vi "Rotating Vectors.vi"() -> ()   [LabVIEW 2019]
uses:
  <vilib>/Analysis/1siggen.llb/Ramp Pattern by Samples.vi
  <vilib>/Analysis/2dsp.llb/Complex FFT.vi
  <vilib>/Analysis/2dsp.llb/Real FFT.vi
  Sub - Arrow Point Calculate.vi
  <vilib>/Analysis/NI_AALPro.lvlib
  <vilib>/Analysis/NI_AALBase.lvlib
panel:
  in  "Message Amplitude":dbl=0.5
  in  "DC Offset":dbl
  in  "RF Frequency":dbl
  in  "Message Frequency":dbl=0.2 step=0.1
  in  "stop":bool
  in  "vi path":path
  in  "Vertical Load Button":bool
  in  "Vertical Pause Button":bool
  in  "Upconvert Baseband":bool=TRUE
  out "Vector Graph":cluster{"z vector":cdb[]}[](graph)=[{"z vector"=[0.0+0.0i, 0.20656463842372266-0.4553361946439979i, 0.21632021300842424-0.355813188436778i, 0.20656463842372266-0.4553361946439979i, 0.12525297407962463-0.3971261161215226i, 0.20656463842372266-0.4553361946439979i]}, {"z vector"=[0.0+0.0i, 0.20656463842372266+0.4553361946439979i, 0.1252529740796247+0.3971261161215225i, 0.20656463842372266+0.4553361946439979i, 0.21632021300842427+0.355813188436778i, 0.20656463842372266+0.4553361946439979i]}, {"z vector"=[0.0+0.0i, 0.4131292768474453+0.0i, 0.32652673646900143+0.05000000000000002i, 0.4131292768474453+0.0i, 0.3265267364690015-0.050000000000000044i, 0.4131292768474453+0.0i]}, {"z vector"=[0.0+0.0i, 0.0+0.0i, nan+nani, 0.0+0.0i, nan+nani, 0.0+0.0i]}, {"z vector"=[0.0+0.0i, 0.4131292768474453+0.0i, 0.32652673646900143+0.05000000000000002i, 0.4131292768474453+0.0i, 0.3265267364690015-0.050000000000000044i, 0.4131292768474453+0.0i]}, {"z vector"=[0.0+0.0i, 0.4131292768474453+0.0i, 0.32652673646900143+0.05000000000000002i, 0.4131292768474453+0.0i, 0.3265267364690015-0.050000000000000044i, 0.4131292768474453+0.0i]}, {"z vector"=[0.4131292768474453+0.0i, 0.4131292768474453+0.0i, nan+nani, 0.4131292768474453+0.0i, nan+nani, 0.4131292768474453+0.0i]}, {"z vector"=[0.0+0.0i, 1.0+0.0i, 0.9133974596215562+0.05000000000000002i, 1.0+0.0i, 0.9133974596215562-0.050000000000000044i, 1.0+0.0i]}]
  out "Time Domain":cluster{dbl, dbl, dbl}(graph)={0.4131292768474453, 0.4131292768474453, 1.0}
  out "Vector Sum Frequency Response":dbl[][](graph)
  out "Individual Vectors":dbl[][](graph)
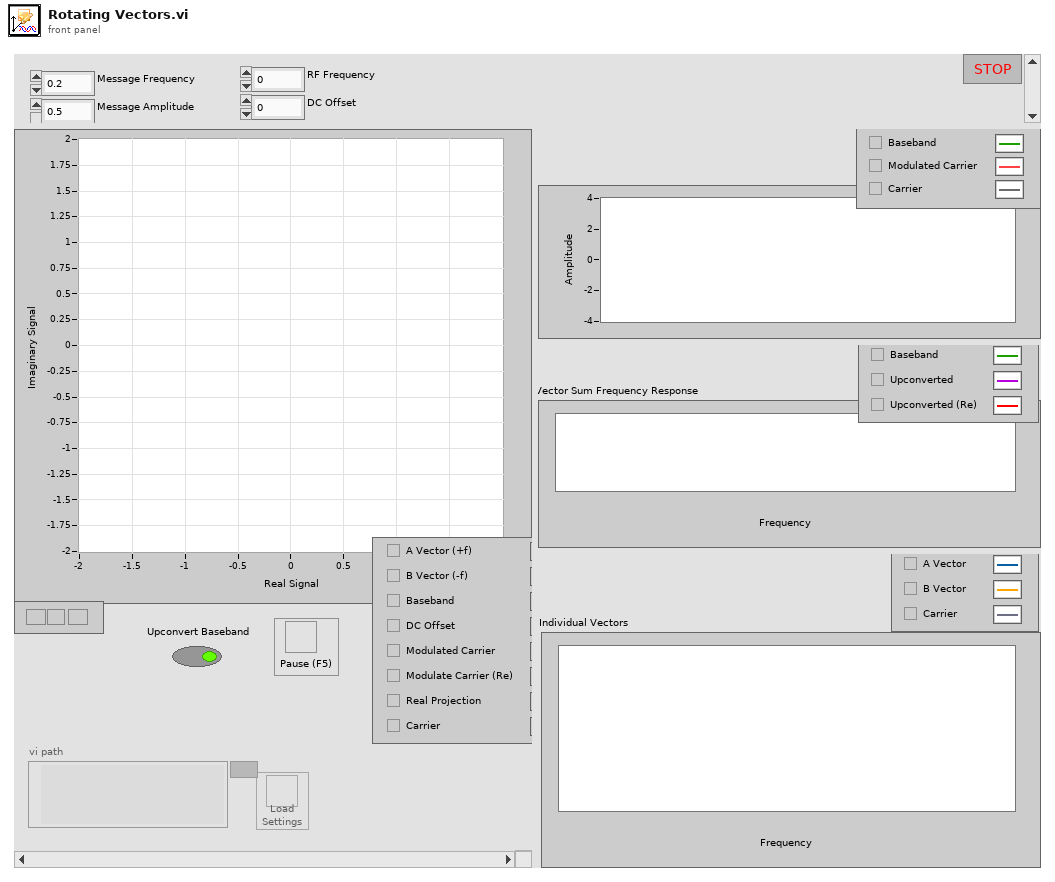
[diagram p1: front panel]
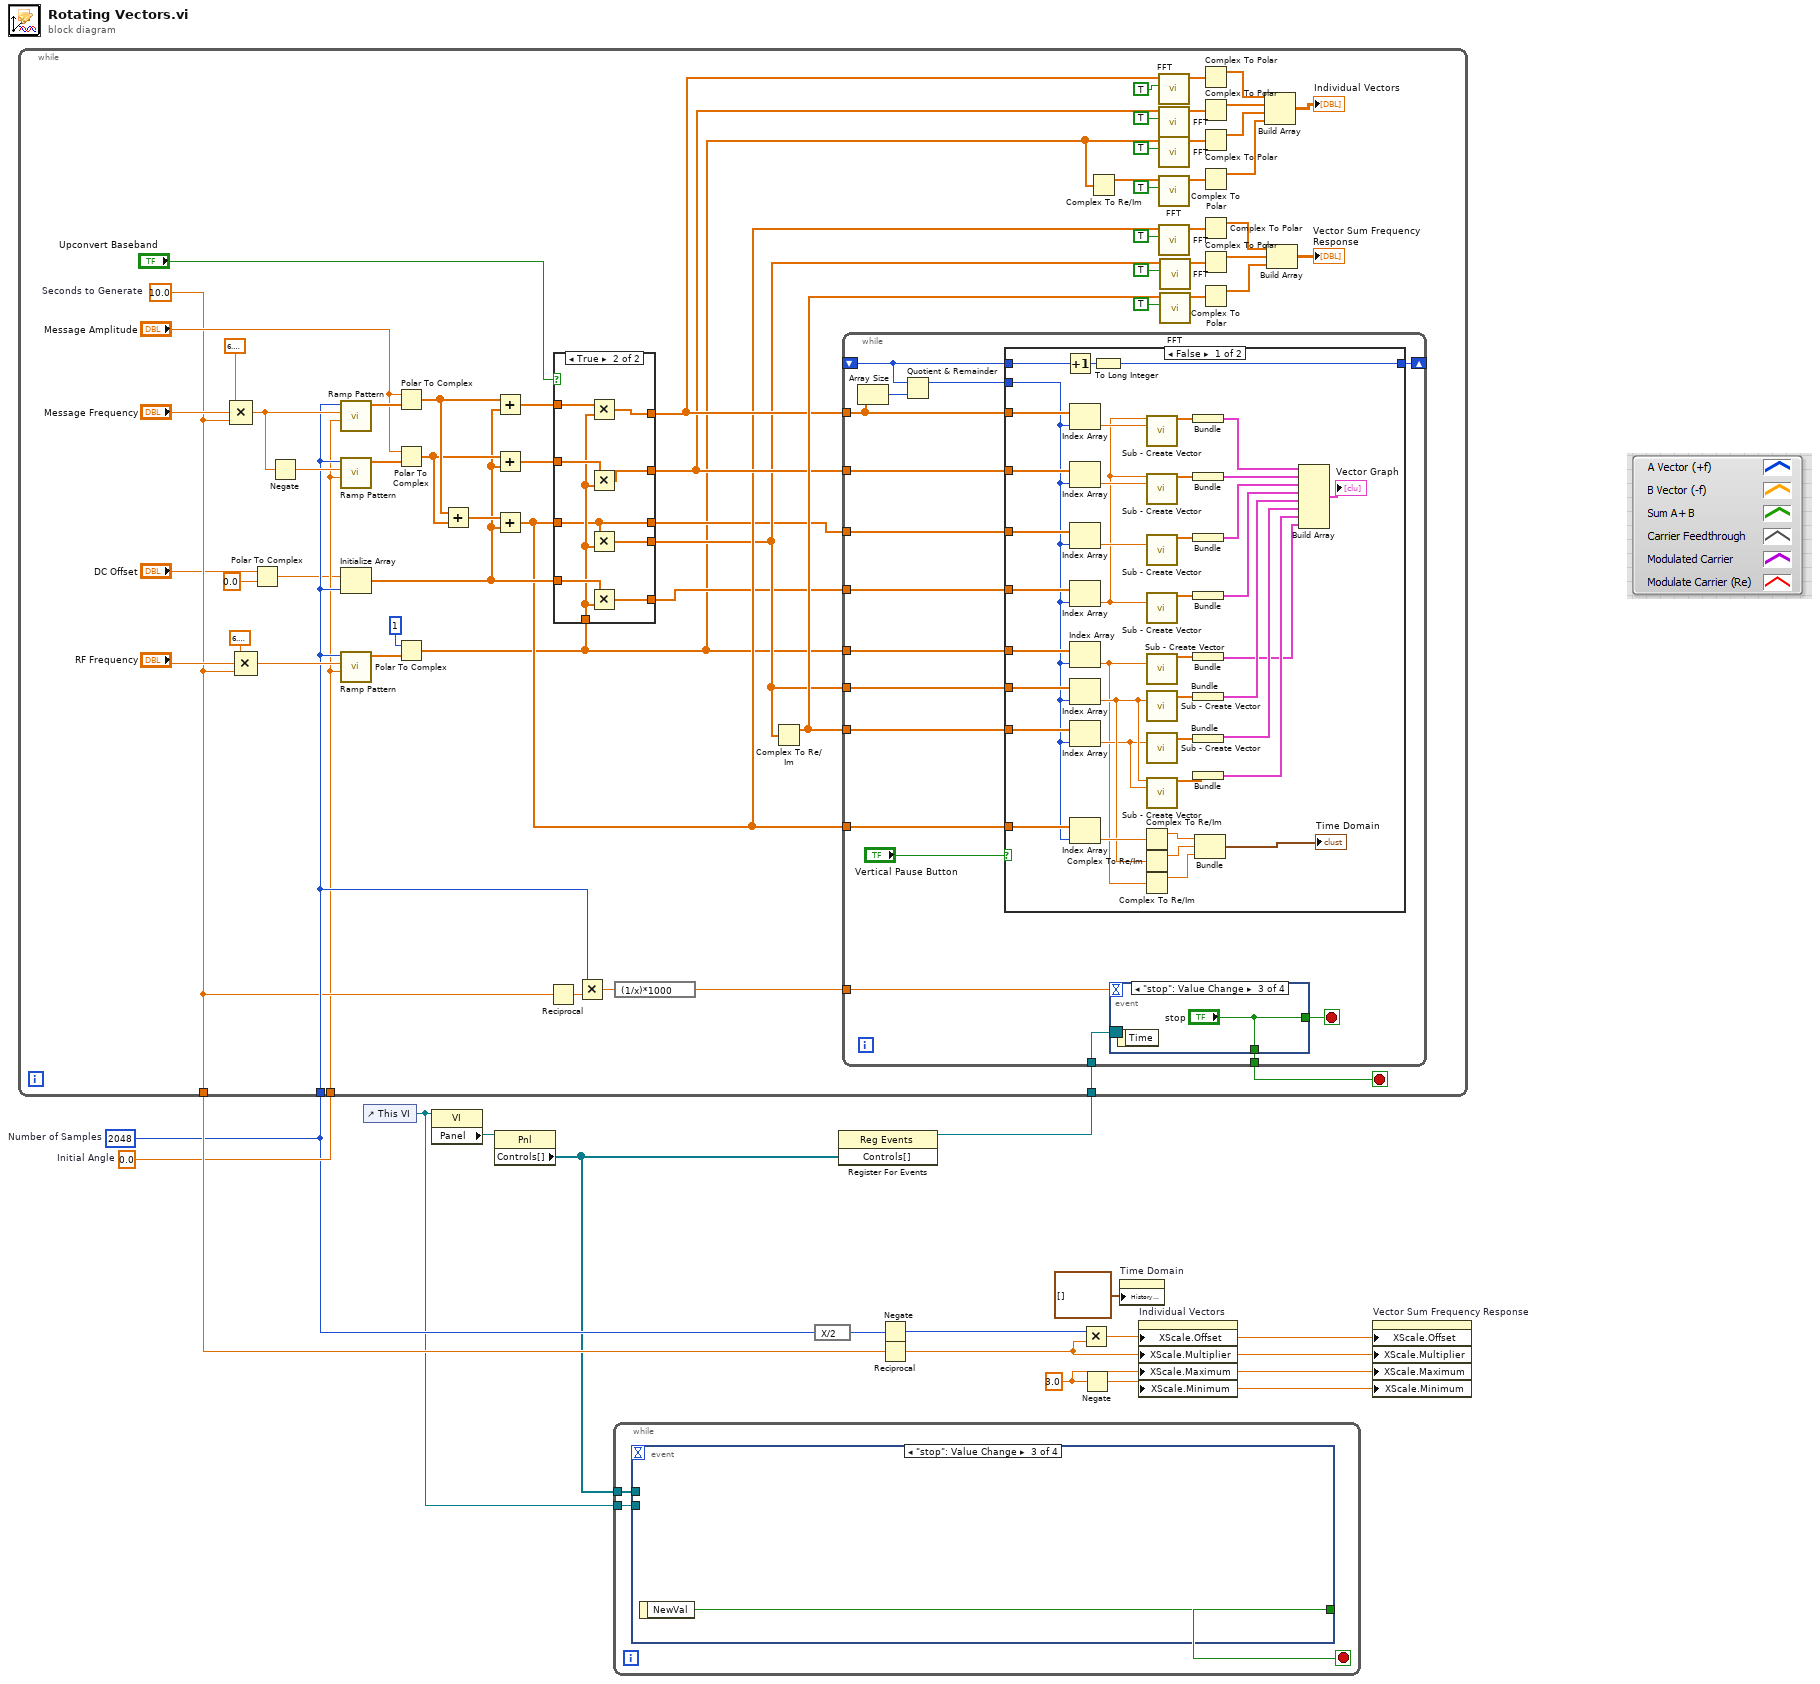
[diagram p0: block diagram]
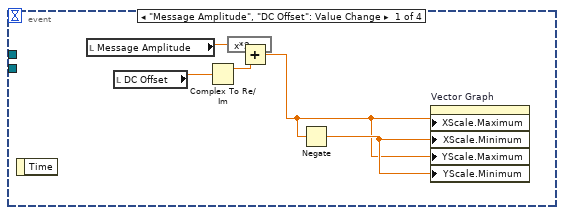
[diagram p2: hidden frame]
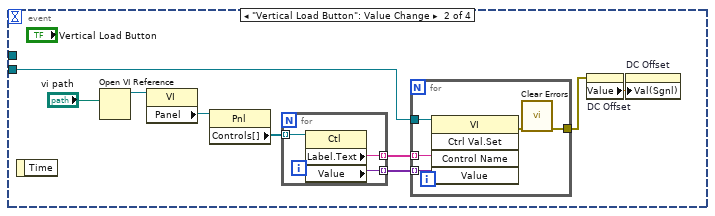
[diagram p3: hidden frame]
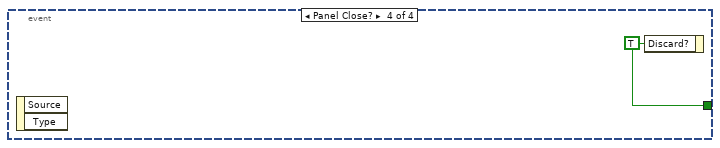
[diagram p4: hidden frame]
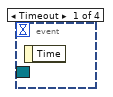
[diagram p7: hidden frame]
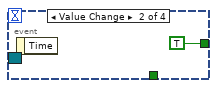
[diagram p8: hidden frame]
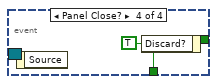
[diagram p9: hidden frame]
diagram:
  w4 = 2048  # Number of Samples
  w5 = 0.0  # Initial Angle
  w11 = 3.0 ("X Scale.Range:Maximum")
  n1 = control-ref of="This VI"() -> (w1:refnum<vi>)
  n2 = property class="VI"(reference=w1) -> ("Panel"=w7:refnum<vi>)  [unwired: 1 in, 2 out]
  n3 = property class="Pnl"(reference=w7) -> ("Controls[]"=w2:refnum<vi>[])  [unwired: 1 in, 2 out]
  n4 = while {
    tunnel: w2 -> [w16]
    tunnel: w1 -> [w15]
    stop <- w17 stop-if-true
    n5 = event shown="[2] \"stop\": Value Change" {
      selector: _ -> [_ _ _ _]
      dyn-events: _ -> [_ _ _ _]
      timeout: _ -> [_ _ _ _]
      tunnel: [_ _ w41 w42] -> w17
      tunnel: w16 -> [_ _ _ _]
      tunnel: w15 -> [_ w29 _ _]
      event "Message Amplitude", "DC Offset": Value Change {
        n6 = event-data() -> ()  [unwired: 1 in, 1 out]
        n7 = local read "Message Amplitude"() -> (w21:dbl)
        n8 = local read "DC Offset"() -> (w22:dbl)
        n9 = Complex To Re/Im(x + iy=w22) -> (x=w19:dbl)  [unwired: 1 out]
        n10 = expression code="x*2"(w21) -> (w18:dbl)
        n11 = Add(x=w18, y=w19) -> (x+y=w20:dbl)
        n12 = Negate(x=w20) -> (-x=w23:dbl)
        n13 = property on="Vector Graph" class="XYGraph (strict)"("XScale.Maximum"=w20, "XScale.Minimum"=w23, "YScale.Maximum"=w20, "YScale.Minimum"=w23) -> ()  [unwired: 2 in, 2 out]
      }
      event "Vertical Load Button": Value Change {
        n14 = event-data() -> ()  [unwired: 1 in, 1 out]
        n15 = Open VI Reference(vi path="vi path") -> (vi reference=w31:refnum<vi>)  [unwired: 5 in, 1 out]
        n16 = property class="VI"(reference=w31) -> ("Panel"=w32:refnum<vi>)  [unwired: 1 in, 2 out]
        n17 = property class="Pnl"(reference=w32) -> ("Controls[]"=w30:refnum<vi>[])  [unwired: 1 in, 2 out]
        n18 = for {
          tunnel: w30 -> [w40] mode=indexing
          tunnel: [w39] -> w28 mode=indexing
          tunnel: [w38] -> w27 mode=indexing
          n19 = property class="Ctl"(reference=w40) -> ("Label.Text"=w39:string, "Value"=w38:variant)  [unwired: 1 in, 2 out]
        }
        n20 = for {
          tunnel: w29 -> [w37]
          tunnel: w28 -> [w36] mode=indexing
          tunnel: w27 -> [w35] mode=indexing
          tunnel: [w33] -> w24
          n21 = invoke class="VI" method="Ctrl Val.Set"(reference=w37, "Control Name"=w36, "Value"=w35) -> (error out=w34:errorcluster)  [unwired: 2 in, 4 out]
          n22 = call <vilib>:"Clear Errors.vi"("error in (no error)"=w34) -> ("error out"=w33:errorcluster)  [unwired: 5 in, 1 out]
        }
        n23 = property on="DC Offset" class="DigNum (strict)"(error in=w24) -> ("Value"=w25:dbl)  [unwired: 1 in, 2 out]
        n24 = property on="DC Offset" class="DigNum (strict)"("Val(Sgnl)"=w25) -> ()  [unwired: 2 in, 2 out]
      }
      event "stop": Value Change {
        n25 = event-data() -> ("NewVal"=w41:bool)  [unwired: 1 in]
      }
      event Panel Close? {
        w42 = TRUE ("Discard?")
        n26 = event-data() -> ()  [unwired: 1 in, 2 out]
        n27 = event-data("Discard?"=w42) -> ()  [unwired: 1 in, 1 out]
      }
    }
  }
  n28 = expression code="X/2"(w4) -> (w13:i32)
  n29 = register-events(w2) -> (reference out=w6:refnum<event-registration>)  [unwired: 2 in, 1 out]
  n30 = while {
    tunnel: [w72] -> w8
    tunnel: w4 -> [w76]
    tunnel: w6 -> [w75]
    tunnel: w5 -> [w65]
    stop <- w73 stop-if-true
    w72 = 10.0  # Seconds to Generate
    n31 = Compound Arithmetic op=MULTIPLY(6.283185307179586, "Message Frequency", w72) -> (w85:dbl)
    n32 = Compound Arithmetic op=MULTIPLY(6.283185307179586, "RF Frequency", w72) -> (w79:dbl)
    n33 = Polar To Complex(1:0.0 ("theta"), 2:"DC Offset") -> (0:w51:cdb)
    n34 = Negate(x=w85) -> (-x=w87:dbl)
    n35 = call-poly <vilib>:"Ramp Pattern.vi"("start"=w65, "end"=w85, "samples"=w76) -> ("Ramp Pattern"=w98:dbl[])  [unwired: 7 in, 1 out]
    n36 = call-poly <vilib>:"Ramp Pattern.vi"("start"=w65, "end"=w87, "samples"=w76) -> ("Ramp Pattern"=w88:dbl[])  [unwired: 7 in, 1 out]
    n37 = Initialize Array(w51, w76) -> (w55:cdb[])
    n38 = call-poly <vilib>:"Ramp Pattern.vi"("start"=w65, "end"=w79, "samples"=w76) -> ("Ramp Pattern"=w86:dbl[])  [unwired: 7 in, 1 out]
    n39 = Polar To Complex(1:w98, 2:"Message Amplitude") -> (0:w78:cdb[])
    n40 = Polar To Complex(1:w88, 2:"Message Amplitude") -> (0:w77:cdb[])
    n41 = Polar To Complex(1:w86, 2:1) -> (0:w45:cdb[])
    n42 = Add(x=w78, y=w77) -> (x+y=w66:cdb[])
    n43 = Add(x=w78, y=w55) -> (x+y=w60:cdb[])
    n44 = Add(x=w77, y=w55) -> (x+y=w59:cdb[])
    n45 = Add(x=w66, y=w55) -> (x+y=w54:cdb[])
    n46 = Reciprocal(x=w72) -> (1/x=w96:dbl)
    n47 = case shown="True" "Upconvert Baseband" {
      tunnel: w60 -> [w106 w117]
      tunnel: w59 -> [w107 w116]
      tunnel: w55 -> [w108 w115]
      tunnel: w54 -> [w105 w109]
      tunnel: w45 -> [_ w114]
      tunnel: [w108 w113] -> w48
      tunnel: [w105 w112] -> w53
      tunnel: [w107 w111] -> w56
      tunnel: [w106 w110] -> w57
      tunnel: [w105 w109] -> w49
      frame False {
      }
      frame True {
        n48 = Multiply(x=w117, y=w114) -> (x*y=w110:cdb[])
        n49 = Multiply(x=w116, y=w114) -> (x*y=w111:cdb[])
        n50 = Multiply(x=w109, y=w114) -> (x*y=w112:cdb[])
        n51 = Multiply(x=w115, y=w114) -> (x*y=w113:cdb[])
      }
    }
    n52 = Multiply(x=w76, y=w96) -> (x*y=w97:dbl)
    n53 = expression code="(1/x)*1000"(w97) -> (w104:dbl)
    n54 = Complex To Re/Im(x + iy=w53) -> (x=w61:dbl[])  [unwired: 1 out]
    n55 = while {
      tunnel: w57 -> [w125]
      tunnel: w104 -> [w130]
      tunnel: w56 -> [w134]
      tunnel: w49 -> [w133]
      tunnel: w53 -> [w132]
      tunnel: w48 -> [w131]
      tunnel: w75 -> [w126]
      tunnel: [w128] -> w73
      tunnel: w61 -> [w127]
      tunnel: w54 -> [w123]
      shift-right: [w120] -> _
      shift-left: _ -> [w121]
      tunnel: w45 -> [w118]
      stop <- w129 stop-if-true
      n56 = Array Size(array=w125) -> (size(s)=w124:i32)
      n57 = Quotient & Remainder(x=w121, y=w124) -> (x-y*floor(x/y)=w122:i32)  [unwired: 1 out]
      n58 = case shown="False" "Vertical Pause Button" {
        tunnel: w134 -> [w172 _]
        tunnel: w133 -> [w167 _]
        tunnel: w132 -> [w166 _]
        tunnel: w131 -> [w161 _]
        tunnel: w127 -> [w158 _]
        tunnel: w125 -> [w156 _]
        tunnel: w123 -> [w151 _]
        tunnel: w122 -> [w137 _]
        tunnel: w121 -> [w147 w176]
        tunnel: [w146 w176] -> w120
        tunnel: w118 -> [w139 _]
        frame False {
          n59 = Increment(x=w147) -> (x+1=w145:i32)
          n60 = Index Array(array=w156, index=w137) -> (element=w153:cdb)
          n61 = Index Array(array=w172, index=w137) -> (element=w154:cdb)
          n62 = Index Array(array=w167, index=w137) -> (element=w155:cdb)
          n63 = Index Array(array=w161, index=w137) -> (element=w152:cdb)
          n64 = Index Array(array=w139, index=w137) -> (element=w136:cdb)
          n65 = Index Array(array=w166, index=w137) -> (element=w142:cdb)
          n66 = Index Array(array=w158, index=w137) -> (element=w141:dbl)
          n67 = Index Array(array=w151, index=w137) -> (element=w150:cdb)
          n68 = To Long Integer(number=w145) -> (32bit integer=w146:i32)
          n69 = Complex To Re/Im(x + iy=w150) -> (x=w165:dbl)  [unwired: 1 out]
          n70 = Complex To Re/Im(x + iy=w142) -> (x=w164:dbl)  [unwired: 1 out]
          n71 = Complex To Re/Im(x + iy=w136) -> (x=w135:dbl)  [unwired: 1 out]
          n72 = call "Sub - Create Vector.vi"("Vector Start (0 +0i)"=w152, "Vector End"=w153) -> ("Vector Points"=w171:cdb[])  [unwired: 13 in]
          n73 = call "Sub - Create Vector.vi"("Vector Start (0 +0i)"=w152, "Vector End"=w154) -> ("Vector Points"=w170:cdb[])  [unwired: 13 in]
          n74 = call "Sub - Create Vector.vi"("Vector End"=w155) -> ("Vector Points"=w168:cdb[])  [unwired: 14 in]
          n75 = call "Sub - Create Vector.vi"("Vector End"=w152) -> ("Vector Points"=w162:cdb[])  [unwired: 14 in]
          n76 = call "Sub - Create Vector.vi"("Vector End"=w136) -> ("Vector Points"=w140:cdb[])  [unwired: 14 in]
          n77 = call "Sub - Create Vector.vi"("Vector End"=w142) -> ("Vector Points"=w159:cdb[])  [unwired: 14 in]
          n78 = call "Sub - Create Vector.vi"("Vector End"=w141) -> ("Vector Points"=w157:cdb[])  [unwired: 14 in]
          n79 = call "Sub - Create Vector.vi"("Vector Start (0 +0i)"=w142, "Vector End"=w141) -> ("Vector Points"=w144:cdb[])  [unwired: 13 in]
          n80 = Bundle("Vector Points"=w171) -> (w175:cluster{"Vector Points":cdb[]})  [unwired: 1 in]
          n81 = Bundle("Vector Points"=w170) -> (w173:cluster{"Vector Points":cdb[]})  [unwired: 1 in]
          n82 = Bundle("Vector Points"=w168) -> (w169:cluster{"Vector Points":cdb[]})  [unwired: 1 in]
          n83 = Bundle("Vector Points"=w162) -> (w160:cluster{"Vector Points":cdb[]})  [unwired: 1 in]
          n84 = Bundle("Vector Points"=w140) -> (w138:cluster{"Vector Points":cdb[]})  [unwired: 1 in]
          n85 = Bundle("Vector Points"=w159) -> (w149:cluster{"Vector Points":cdb[]})  [unwired: 1 in]
          n86 = Bundle("Vector Points"=w157) -> (w148:cluster{"Vector Points":cdb[]})  [unwired: 1 in]
          n87 = Bundle("Vector Points"=w144) -> (w143:cluster{"Vector Points":cdb[]})  [unwired: 1 in]
          n88 = Bundle(w165, w164, w135) -> (→"Time Domain":cluster{dbl, dbl, dbl})  [unwired: 1 in]
          n89 = Build Array(w175, w173, w169, w160, w149, w148, w143, w138) -> (→"Vector Graph":cluster{"Vector Points":cdb[]}[])
        }
        frame True {
        }
      }
      n90 = event shown="[2] \"stop\": Value Change" {
        selector: w126 -> [_ _ _ _]
        dyn-events: _ -> [_ _ _ _]
        timeout: w130 -> [_ _ _ _]
        tunnel: [_ TRUE "stop" w179] -> w129
        tunnel: [_ _ "stop" w179] -> w128
        event Timeout {
          n91 = event-data() -> ()  [unwired: 1 in, 1 out]
        }
        event Value Change {
          n92 = event-data() -> ()  [unwired: 1 in, 1 out]
        }
        event "stop": Value Change {
          n93 = event-data() -> ()  [unwired: 1 in, 1 out]
        }
        event Panel Close? {
          w179 = TRUE ("Discard?")
          n94 = event-data() -> ()  [unwired: 1 in, 1 out]
          n95 = event-data("Discard?"=w179) -> ()  [unwired: 1 in, 1 out]
        }
      }
    }
    n96 = Complex To Re/Im(x + iy=w45) -> (x=w44:dbl[])  [unwired: 1 out]
    n97 = call-poly <vilib>:"FFT.vi"("shift?"=TRUE, "X"=w57) -> ("FFT {X}"=w102:cdb[])  [unwired: 8 in, 1 out]
    n98 = call-poly <vilib>:"FFT.vi"("shift?"=TRUE, "X"=w56) -> ("FFT {X}"=w95:cdb[])  [unwired: 8 in, 1 out]
    n99 = call-poly <vilib>:"FFT.vi"("shift?"=TRUE, "X"=w45) -> ("FFT {X}"=w69:cdb[])  [unwired: 8 in, 1 out]
    n100 = call-poly <vilib>:"FFT.vi"("shift?"=TRUE, "X"=w44) -> ("FFT {X}"=w47:cdb[])  [unwired: 8 in, 1 out]
    n101 = call-poly <vilib>:"FFT.vi"("shift?"=TRUE, "X"=w54) -> ("FFT {X}"=w90:cdb[])  [unwired: 8 in, 1 out]
    n102 = call-poly <vilib>:"FFT.vi"("shift?"=TRUE, "X"=w53) -> ("FFT {X}"=w83:cdb[])  [unwired: 8 in, 1 out]
    n103 = call-poly <vilib>:"FFT.vi"("shift?"=TRUE, "X"=w61) -> ("FFT {X}"=w63:cdb[])  [unwired: 8 in, 1 out]
    n104 = Complex To Polar(r * e^(i*theta)=w102) -> (r=w99:dbl[])  [unwired: 1 out]
    n105 = Complex To Polar(r * e^(i*theta)=w95) -> (r=w92:dbl[])  [unwired: 1 out]
    n106 = Complex To Polar(r * e^(i*theta)=w69) -> (r=w68:dbl[])  [unwired: 1 out]
    n107 = Complex To Polar(r * e^(i*theta)=w47) -> (r=w43:dbl[])  [unwired: 1 out]
    n108 = Complex To Polar(r * e^(i*theta)=w90) -> (r=w89:dbl[])  [unwired: 1 out]
    n109 = Complex To Polar(r * e^(i*theta)=w83) -> (r=w81:dbl[])  [unwired: 1 out]
    n110 = Complex To Polar(r * e^(i*theta)=w63) -> (r=w62:dbl[])  [unwired: 1 out]
    n111 = Build Array(w99, w92, w68, w43) -> (→"Individual Vectors":dbl[][])
    n112 = Build Array(w89, w81, w62) -> (→"Vector Sum Frequency Response":dbl[][])
  }
  n113 = Negate(x=w13) -> (-x=w14:i32)
  n114 = Reciprocal(x=w8) -> (1/x=w10:dbl)
  n115 = Multiply(x=w14, y=w10) -> (x*y=w9:dbl)
  n116 = Negate(x=w11) -> (-x=w12:dbl)
  n117 = property on="Time Domain" class="WFChart (strict)"("History Data"=cluster{dbl, dbl, dbl}[] []) -> ()  [unwired: 2 in, 2 out]
  n118 = property on="Individual Vectors" class="WFGraph (strict)"("XScale.Offset"=w9, "XScale.Multiplier"=w10, "XScale.Maximum"=w11, "XScale.Minimum"=w12) -> ()  [unwired: 2 in, 2 out]
  n119 = property on="Vector Sum Frequency Response" class="WFGraph (strict)"("XScale.Offset"=w9, "XScale.Multiplier"=w10, "XScale.Maximum"=w11, "XScale.Minimum"=w12) -> ()  [unwired: 2 in, 2 out]
